vi "PartsTracking Controller_Create.vi"(0 "reference in":refnum<class "PartsTracking Controller.lvclass">, 5 "error in (no error)":errorcluster) -> (14 "reference out":refnum<class "PartsTracking Controller.lvclass">, 19 "error out":errorcluster)   [LabVIEW 2015, in "PartsTracking Controller.lvclass"]
doc: "Constructor."
uses:
  PartsTracking Controller.lvclass
  <vilib>/addons/_AddQ/G#Object/G#Object.lvclass
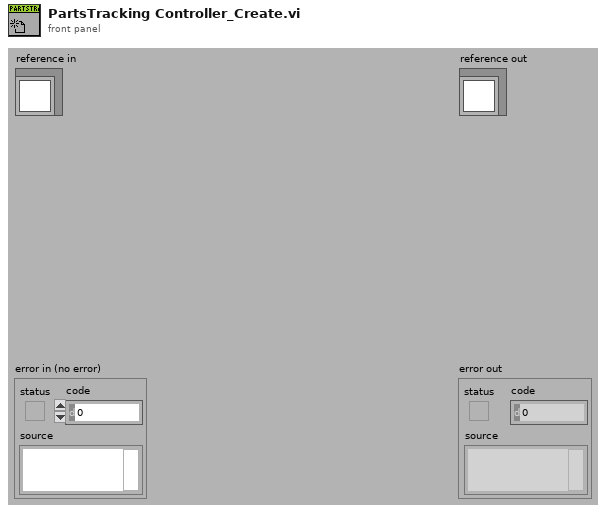
[diagram p1: front panel]
types:
  T1 = typedef "PartsTracking Controller.lvclass/ClassAttributesRef.ctl" = refnum<data-value>
  T2 = typedef "PartsTracking Controller.lvclass/ClassAttributes.ctl" = cluster{"Dummy":bool, "partstracking_controller_ref":refnum<class "PartsTracking Controller.lvclass">}
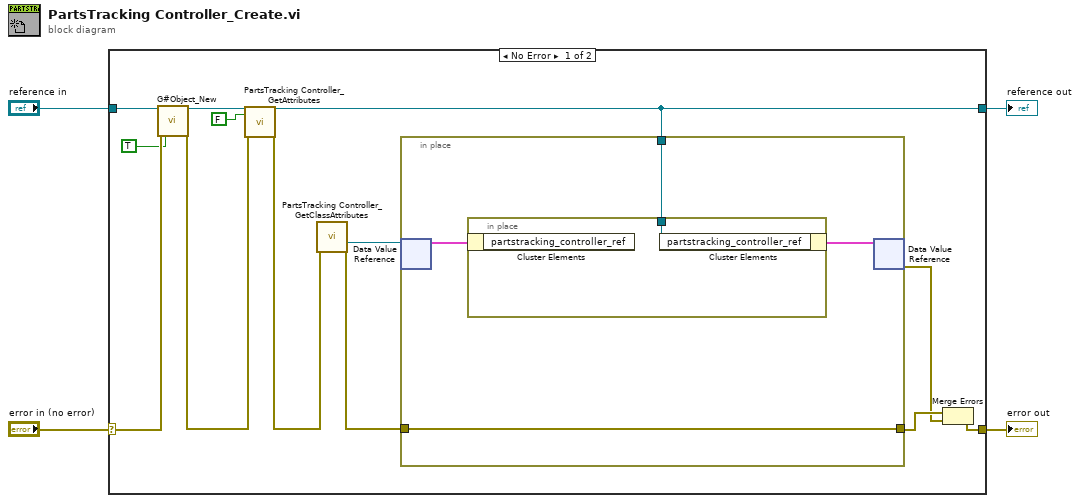
[diagram p0: block diagram]
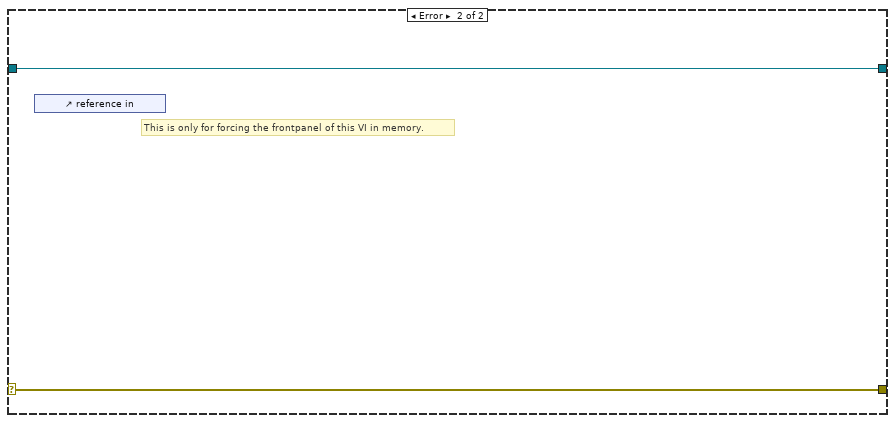
[diagram p2: hidden frame]
diagram:
  n1 = case shown="No Error" "error in (no error)" {
    selector: "error in (no error)" -> [w16 w24]
    tunnel: [w15 w24] -> w3
    tunnel: [w7 w23] -> w1
    tunnel: "reference in" -> [w17 w23]
    frame No Error {
      n2 = call <vilib>:"G#Object_New.vi"("reference in"=w17, "error in (no error)"=w16, "user counter (T)?"=TRUE ("User Counter")) -> ("reference out"=w11:refnum<class "PartsTracking Controller.lvclass">, "error out"=w10:errorcluster)  [unwired: 14 in, 1 out]
      n3 = call "PartsTracking Controller_GetAttributes.vi"("reference in"=w11, "return data? (T)"=FALSE ("return data"), "error in (no error)"=w10) -> ("reference out"=w7:refnum<class "PartsTracking Controller.lvclass">, "error out"=w6:errorcluster)  [unwired: 13 in, 2 out]
      n4 = call "PartsTracking Controller_GetClassAttributes.vi"("error in (no error)"=w6) -> ("class attributes ref"=w8:T1, "error out"=w5:errorcluster)  [unwired: 15 in, 2 out]
      n5 = in-place {
        in-place-border: w5 -> [w19]
        in-place-border: [w19] -> w13
        in-place-border: w7 -> [w18]
        n6 = in-place-dvr #1(w8) -> (w20:T2)  [unwired: 1 out]
        n7 = in-place {
          in-place-border: w18 -> [w22]
          n8 = in-place-cluster #2(w20) -> ()  [unwired: 1 out]
          n9 = in-place-cluster #2("partstracking_controller_ref"=w22) -> (w21:T2)
        }
        n10 = in-place-dvr #1(w21) -> (w12:errorcluster)  [unwired: 1 out]
      }
      n11 = Merge Errors(w13, w12) -> (w15:errorcluster)
    }
    frame Error {
      # "This is only for forcing the frontpanel of this VI in memory."
      n12 = control-ref of="reference in"() -> ()  [unwired: 1 out]
    }
  }
  "error out" <- w3
  "reference out" <- w1
